vi "Update Plot.vi"(8 "error in (no error)":errorcluster, 11 "Lockin Processor in":refnum<class "Lockin Processor.lvclass">) -> (0 "error out":errorcluster, 3 "Lockin Processor out":refnum<class "Lockin Processor.lvclass">)   [LabVIEW 2016, in "Lockin Processor.lvclass"]
uses:
  Lockin Processor.lvclass
  Lockin Processor Configuration.ctl
  Lockin Processor.lvclass/Lockin Processor.ctl
  Read Lockin Processor Configuration.vi
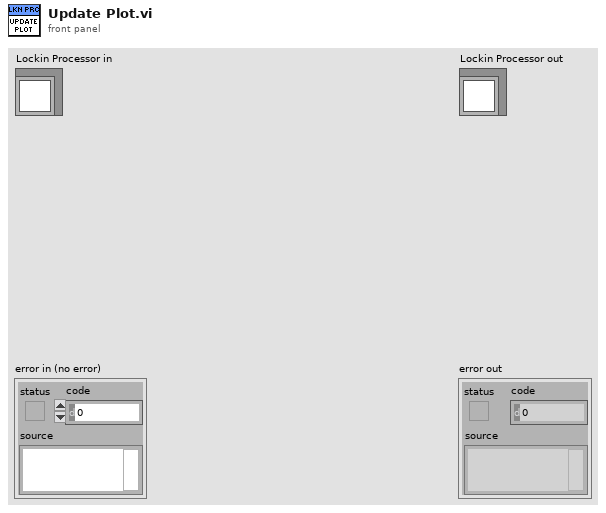
[diagram p1: front panel]
types:
  T1 = typedef "Lockin Processor Configuration.ctl" = cluster{"Time constant":dbl, "Signal channels":string[], "Group":string, "X channel":string, "Live update":bool, "Phases":dbl[], "Harmonics":i32[]}
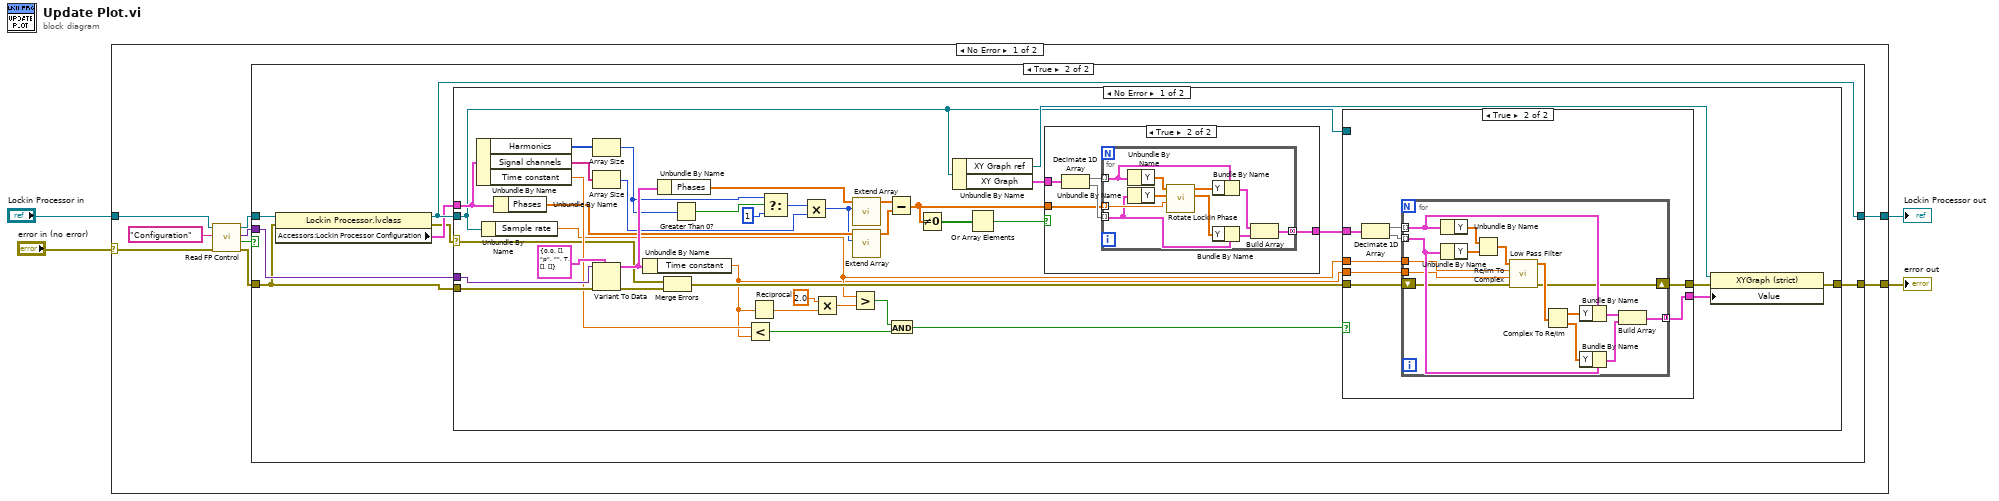
[diagram p0: block diagram]
diagram:
  n1 = case shown="No Error" "error in (no error)" {
    selector: "error in (no error)" -> [w6 w105]
    tunnel: [w5 w105] -> w3
    tunnel: [w7 w104] -> w1
    tunnel: "Lockin Processor in" -> [w8 w104]
    frame No Error {
      n2 = call-dynamic "Read FP Control.vi"("error in (no error)"=w6, "Control Name"="Configuration", "Measure Object in"=w8) -> ("error out"=w11:errorcluster, "Present"=w10:bool, "Control Value"=w12:variant, "Measure Object out"=w9:refnum<class "Lockin Processor.lvclass">)  [unwired: 5 in]
      n3 = case shown="True" w10 {
        tunnel: w12 -> [_ w22]
        tunnel: w11 -> [w14 w20]
        tunnel: w9 -> [w15 w21]
        tunnel: [w15 w18] -> w7
        tunnel: [w14 w19] -> w5
        frame False {
        }
        frame True {
          n4 = property class="Lockin Processor.lvclass"(reference=w21, error in=w20) -> (reference out=w18:refnum<class "Lockin Processor.lvclass">, error out=w16:errorcluster, "Accessors:Lockin Processor Configuration"=w17:T1)
          n5 = case shown="No Error" w16 {
            selector: w16 -> [w49 _]
            tunnel: w22 -> [w61 _]
            tunnel: w20 -> [w59 w103]
            tunnel: [w45 w103] -> w19
            tunnel: w18 -> [w43 _]
            tunnel: w17 -> [w53 _]
            frame No Error {
              n6 = Unbundle By Name(w53) -> ("Harmonics"=w28:i32[], "Signal channels"=w35:string[], "Time constant"=w57:dbl)
              n7 = Unbundle By Name(w43) -> ("Sample rate"=w42:dbl)
              n8 = Unbundle By Name(w53) -> ("Phases"=w33:dbl[])
              n9 = Array Size(array=w28) -> (size(s)=w26:i32)
              n10 = Array Size(array=w35) -> (size(s)=w34:i32)
              n11 = Variant To Data(error in=w59, type=T1 {"Time constant"=0.0, "Signal channels"=[], "Group"="p", "X channel"="", "Live update"=TRUE, "Phases"=[], "Harmonics"=[]} ("Configuration"), Variant=w61) -> (data=w52:T1, error out=w58:errorcluster)
              n12 = Unbundle By Name(w52) -> ("Time constant"=w41:dbl)
              n13 = Unbundle By Name(w52) -> ("Phases"=w32:dbl[])
              n14 = Merge Errors(w49, w58) -> (w54:errorcluster)
              n15 = Greater Than 0?(x=w26) -> (x > 0?=w27:bool)
              n16 = Less?(x=w57, y=w41) -> (x < y?=w56:bool)
              n17 = Reciprocal(x=w41) -> (1/x=w40:dbl)
              n18 = Select(t=w26, s=w27, f=1) -> (s? t:f=w23:i32)
              n19 = Multiply(x=w23, y=w34) -> (x*y=w24:i32)
              n20 = Multiply(x=2.0, y=w40) -> (x*y=w38:dbl)
              n21 = Greater?(x=w42, y=w38) -> (0:w36:bool)
              n22 = call "Extend Array.vi"("Extend to size"=w24, "Array in"=w32) -> ("Array out"=w29:dbl[])  [unwired: 8 in, 1 out]
              n23 = call "Extend Array.vi"("Extend to size"=w24, "Array in"=w33) -> ("Array out"=w30:dbl[])  [unwired: 8 in, 1 out]
              n24 = Subtract(x=w29, y=w30) -> (x-y=w31:dbl[])
              n25 = And(x=w36, y=w56) -> (x .and. y?=w37:bool)
              n26 = Not Equal To 0?(x=w31) -> (x != 0?=w51:bool[])
              n27 = Unbundle By Name(w43) -> ("XY Graph ref"=w48:refnum<vi>, "XY Graph"=w44:cluster{"X":dbl[], "Y":dbl[]}[])
              n28 = Or Array Elements(Boolean array=w51) -> (logical OR=w50:bool)
              n29 = case shown="True" w50 {
                tunnel: w44 -> [w87 w92]
                tunnel: [w87 w89] -> w55
                tunnel: w31 -> [_ w88]
                frame False {
                }
                frame True {
                  n30 = Decimate 1D Array(w92) -> (w91:cluster{"X":dbl[], "Y":dbl[]}[], w90:cluster{"X":dbl[], "Y":dbl[]}[])
                  n31 = for {
                    tunnel: w91 -> [w100] mode=indexing
                    tunnel: w90 -> [w97] mode=indexing
                    tunnel: w88 -> [w101] mode=indexing
                    tunnel: [w95] -> w89 mode=concatenating
                    n32 = Unbundle By Name(w100) -> ("Y"=w93:dbl[])
                    n33 = Unbundle By Name(w97) -> ("Y"=w102:dbl[])
                    n34 = call "Rotate Lockin Phase.vi"("Phase"=w101, "Array Y in"=w102, "Array X in"=w93) -> ("Array Y out"=w98:dbl[], "Array X out"=w99:dbl[])  [unwired: 7 in]
                    n35 = Bundle By Name(cluster=w100, "Y"=w99) -> (w96:cluster{"X":dbl[], "Y":dbl[]})
                    n36 = Bundle By Name(cluster=w97, "Y"=w98) -> (w94:cluster{"X":dbl[], "Y":dbl[]})
                    n37 = Build Array(w96, w94) -> (w95:cluster{"X":dbl[], "Y":dbl[]}[])
                  }
                }
              }
              n38 = case shown="True" w37 {
                tunnel: w55 -> [w63 w71]
                tunnel: w41 -> [_ w68]
                tunnel: [w63 w67] -> w47
                tunnel: w54 -> [w62 w66]
                tunnel: [w62 w65] -> w46
                tunnel: w43 -> [_ _]
                tunnel: w42 -> [_ w64]
                frame False {
                }
                frame True {
                  n39 = Decimate 1D Array(w71) -> (w70:cluster{"X":dbl[], "Y":dbl[]}[], w69:cluster{"X":dbl[], "Y":dbl[]}[])
                  n40 = for {
                    tunnel: w70 -> [w77] mode=indexing
                    tunnel: w69 -> [w76] mode=indexing
                    tunnel: w68 -> [w75]
                    tunnel: [w85] -> w67 mode=concatenating
                    shift-right: [w73] -> w65
                    shift-left: w66 -> [w74]
                    tunnel: w64 -> [w72]
                    n41 = Unbundle By Name(w77) -> ("Y"=w83:dbl[])
                    n42 = Unbundle By Name(w76) -> ("Y"=w82:dbl[])
                    n43 = Re/Im To Complex(1:w82, 2:w83) -> (0:w81:cdb[])
                    n44 = call "Low Pass Filter.vi"("Error In"=w74, "Time constant"=w75, "Sample rate"=w72, "Data"=w81) -> ("Error Out"=w73:errorcluster, "Data out"=w80:cdb[])  [unwired: 6 in]
                    n45 = Complex To Re/Im(x + iy=w80) -> (x=w79:dbl[], y=w78:dbl[])
                    n46 = Bundle By Name(cluster=w77, "Y"=w79) -> (w86:cluster{"X":dbl[], "Y":dbl[]})
                    n47 = Bundle By Name(cluster=w76, "Y"=w78) -> (w84:cluster{"X":dbl[], "Y":dbl[]})
                    n48 = Build Array(w86, w84) -> (w85:cluster{"X":dbl[], "Y":dbl[]}[])
                  }
                }
              }
              n49 = property class="XYGraph (strict)"(reference=w48, error in=w46, "Value"=w47) -> (error out=w45:errorcluster)  [unwired: 1 out]
            }
            frame Error {
            }
          }
        }
      }
    }
    frame Error {
    }
  }
  "error out" <- w3
  "Lockin Processor out" <- w1
